vi "Gather Images.vi"() -> ()   [LabVIEW 2017, in "DocTools.lvlib"]
uses:
  DocTools.lvlib
panel:
  out "Progress":dbl(slide) scale=0.0..1.0
  out "Working Directory (../doc/)":path
  # "Please make sure the .lvlibp is located in a subfolder of your project directory"
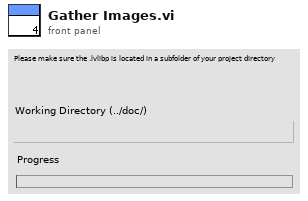
[diagram p1: front panel]
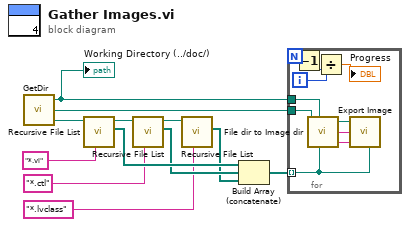
[diagram p0: block diagram]
diagram:
  n1 = call "GetDir.vi"() -> ("Project Directory (../)"=w12:path, "Documentation Directory (../doc/)"=w1:path, "Image Directory (../doc/img/)"=w2:path)
  "Working Directory (../doc/)" <- w2
  n2 = call <vilib>:"Recursive File List.vi"("pattern"="*.vi", "Folder Path"=w12) -> ("All Files in Dir"=w9:path[], "dup Folder Path"=w11:path)  [unwired: 5 in, 3 out]
  n3 = call <vilib>:"Recursive File List.vi"("pattern"="*.ctl", "Folder Path"=w11) -> ("All Files in Dir"=w8:path[], "dup Folder Path"=w10:path)  [unwired: 5 in, 3 out]
  n4 = call <vilib>:"Recursive File List.vi"("pattern"="*.lvclass", "Folder Path"=w10) -> ("All Files in Dir"=w7:path[])  [unwired: 5 in, 4 out]
  n5 = Build Array (concatenate)(w9, w8, w7) -> (w3:path[])
  n6 = for {
    N -> [w17]
    tunnel: w3 -> [w19] mode=indexing
    tunnel: w2 -> [w14]
    tunnel: w1 -> [w13]
    i -> [w18]
    n7 = Decrement(x=w17) -> (x-1=w15:i32)
    n8 = call "File dir to Image dir.vi"("Documentation Folder"=w13, "Image Folder"=w14, "File"=w19) -> ("Folder"=w22:path, "File"=w21:string, "Type"=w20:string)  [unwired: 4 in]
    n9 = Divide(x=w18, y=w15) -> (x/y=→"Progress":dbl)
    n10 = call "Export Image.vi"("Image Folder"=w22, "Filename"=w21, "Type"=w20, "File Directory"=w19) -> ()  [unwired: 6 in]
  }
